vi "4.3 Arguments - Safe Arguments if it contains key words of CSM.vi"() -> ()   [LabVIEW 2017]
doc: "### 4.3 Arguments - Safe Arguments if it contains key words of CSM.vi\n\n#### Overview\nDemonstrates how to convert reserved CSM keywords in an argument string to a HEXSTR (0-9, A-F) format and how to convert back to original form to prevent affecting parsing of CSM message strings.\n\n#### Introduction\nThis example demonstrates how to convert reserved CSM keywords in an argument string to a %HEXSTR (0-9, A-F) format and how to convert back to original form to prevent affecting parsing of CSM message strings."
uses:
  user.lib/_NEVSTOP/Communicable State Machine(CSM)/AdvanceAPI/CSM - Keywords.vi
  user.lib/_NEVSTOP/Communicable State Machine(CSM)/Communicable State Machine.lvlib
panel:
  in  "Argument String 3":string="https://github.com/NEVSTOP-LAB/Communicable-State-Machine"
  out "Safe Argument String 3":string="https:%2F%2Fgithub.com/NEVSTOP-LAB/Communicable-State-Machine"
  out "Safe Argument String 2":string="c:\\abc\\def.txt"
  in  "Argument String 2":string="c:\\abc\\def.txt"
  out "Safe Argument String":string="eaasdf%2D%3Efqwvrf%2D%26#%0Adddd\\\\\\\\\\not comments%0A%2F%2Fadcd\\\\de/assfd%0A%2C %5B%3B%5D%0A%2D%40asdfvq%3C%2D1234"
  out "Origin Argument String":string="eaasdf->fqwvrf-&#\ndddd\\\\\\\\\\not comments\n//adcd\\\\de/assfd\n, [;]\n-@asdfvq<-1234"
  in  "Argument String":string="eaasdf->fqwvrf-&#\ndddd\\\\\\\\\\not comments\n//adcd\\\\de/assfd\n, [;]\n-@asdfvq<-1234"
  # "#CSM-Example Overview\nDemonstrates how to convert reserved CSM keywords in an argument string to a HEXSTR (0-9, A-F) format and how to convert back to original form to prevent affecting parsing of CSM message strings."
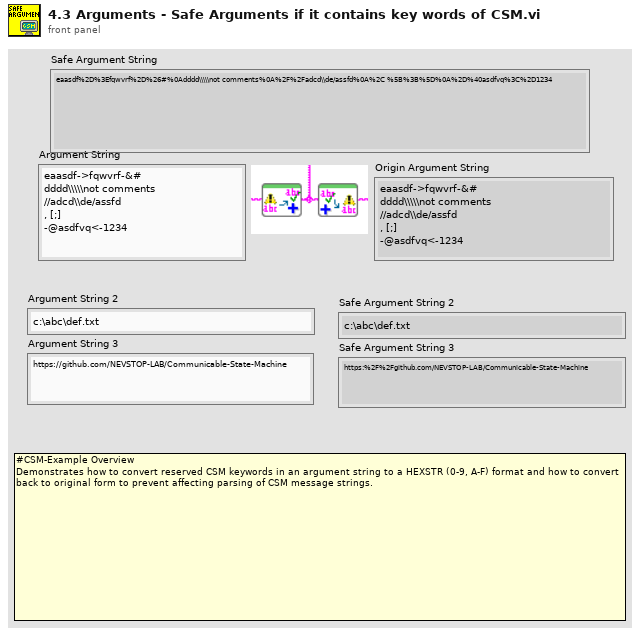
[diagram p1: front panel]
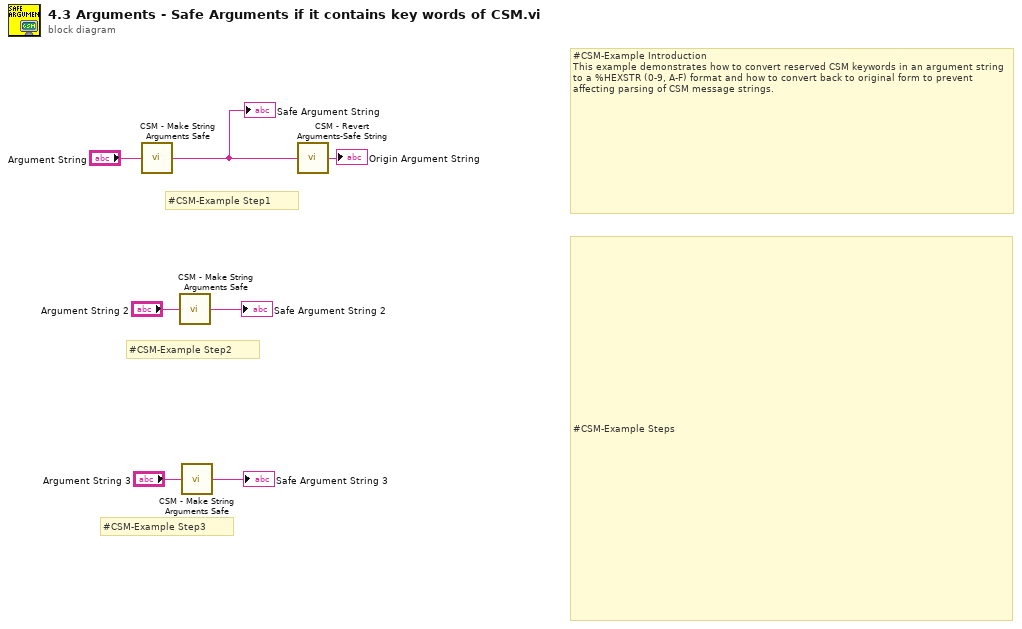
[diagram p0: block diagram]
diagram:
  # "#CSM-Example Step1"
  # "#CSM-Example Step2"
  # "#CSM-Example Step3"
  # "#CSM-Example Steps"
  # "#CSM-Example Introduction\nThis example demonstrates how to convert reserved CSM keywords in an argument string to a %HEXSTR (0-9, A-F) format and how to convert back to original form to prevent affecting parsing of CSM message strings."
  n1 = call "CSM - Make String Arguments Safe.vi"("Argument String"="Argument String") -> ("Safe Argument String"=w1:string)  [unwired: 8 in]
  "Safe Argument String" <- w1
  n2 = call "CSM - Make String Arguments Safe.vi"("Argument String"="Argument String 2") -> ("Safe Argument String"=→"Safe Argument String 2":string)  [unwired: 8 in]
  n3 = call "CSM - Make String Arguments Safe.vi"("Argument String"="Argument String 3") -> ("Safe Argument String"=→"Safe Argument String 3":string)  [unwired: 8 in]
  n4 = call "CSM - Revert Arguments-Safe String.vi"("Safe Argument String"=w1) -> ("Origin Argument String"=→"Origin Argument String":string)  [unwired: 8 in]
